vi "Select Comms Method.vi"(8 "Error In":errorcluster) -> (0 "Error Out":errorcluster, 3 "User DOne":bool)   [LabVIEW 2014]
uses:
  Application Support/Stop Button/SubVI/Get Stop Button Status.vi
  Application Support/Front Panel/Window In Front/Bring Caller to Front.vi
  Settings File/SubVI/Load Connection Type.vi
  Settings File/SubVI/Load Serial Baud Rate.vi
  Settings File/SubVI/Save Connection Type.vi
  Settings File/SubVI/Save Baud Rate.vi
  Controls/Telemetry Connection Type.ctl
  Aircraft Information/Sub VI/Set Aircraft Information.vi
  Aircraft Information/Controls/Aircraft Mode.ctl
  Aircraft Information/Controls/Base Mode.ctl
  Aircraft Information/Controls/Drone Information.ctl
  Controls/Telemetry Serial Baud Rate.ctl
  GUI Design/Buttons/Standard button.ctl
panel:
  in  "VISA resource name":refnum<visa-resource-name>
  in  "Baud Rate":T1=enum."115200"
  in  "Connection Type":T2
  out "String":string="COMMUNICATION METHOD"
  in  "Done":T3
  in  "Join Mission":bool
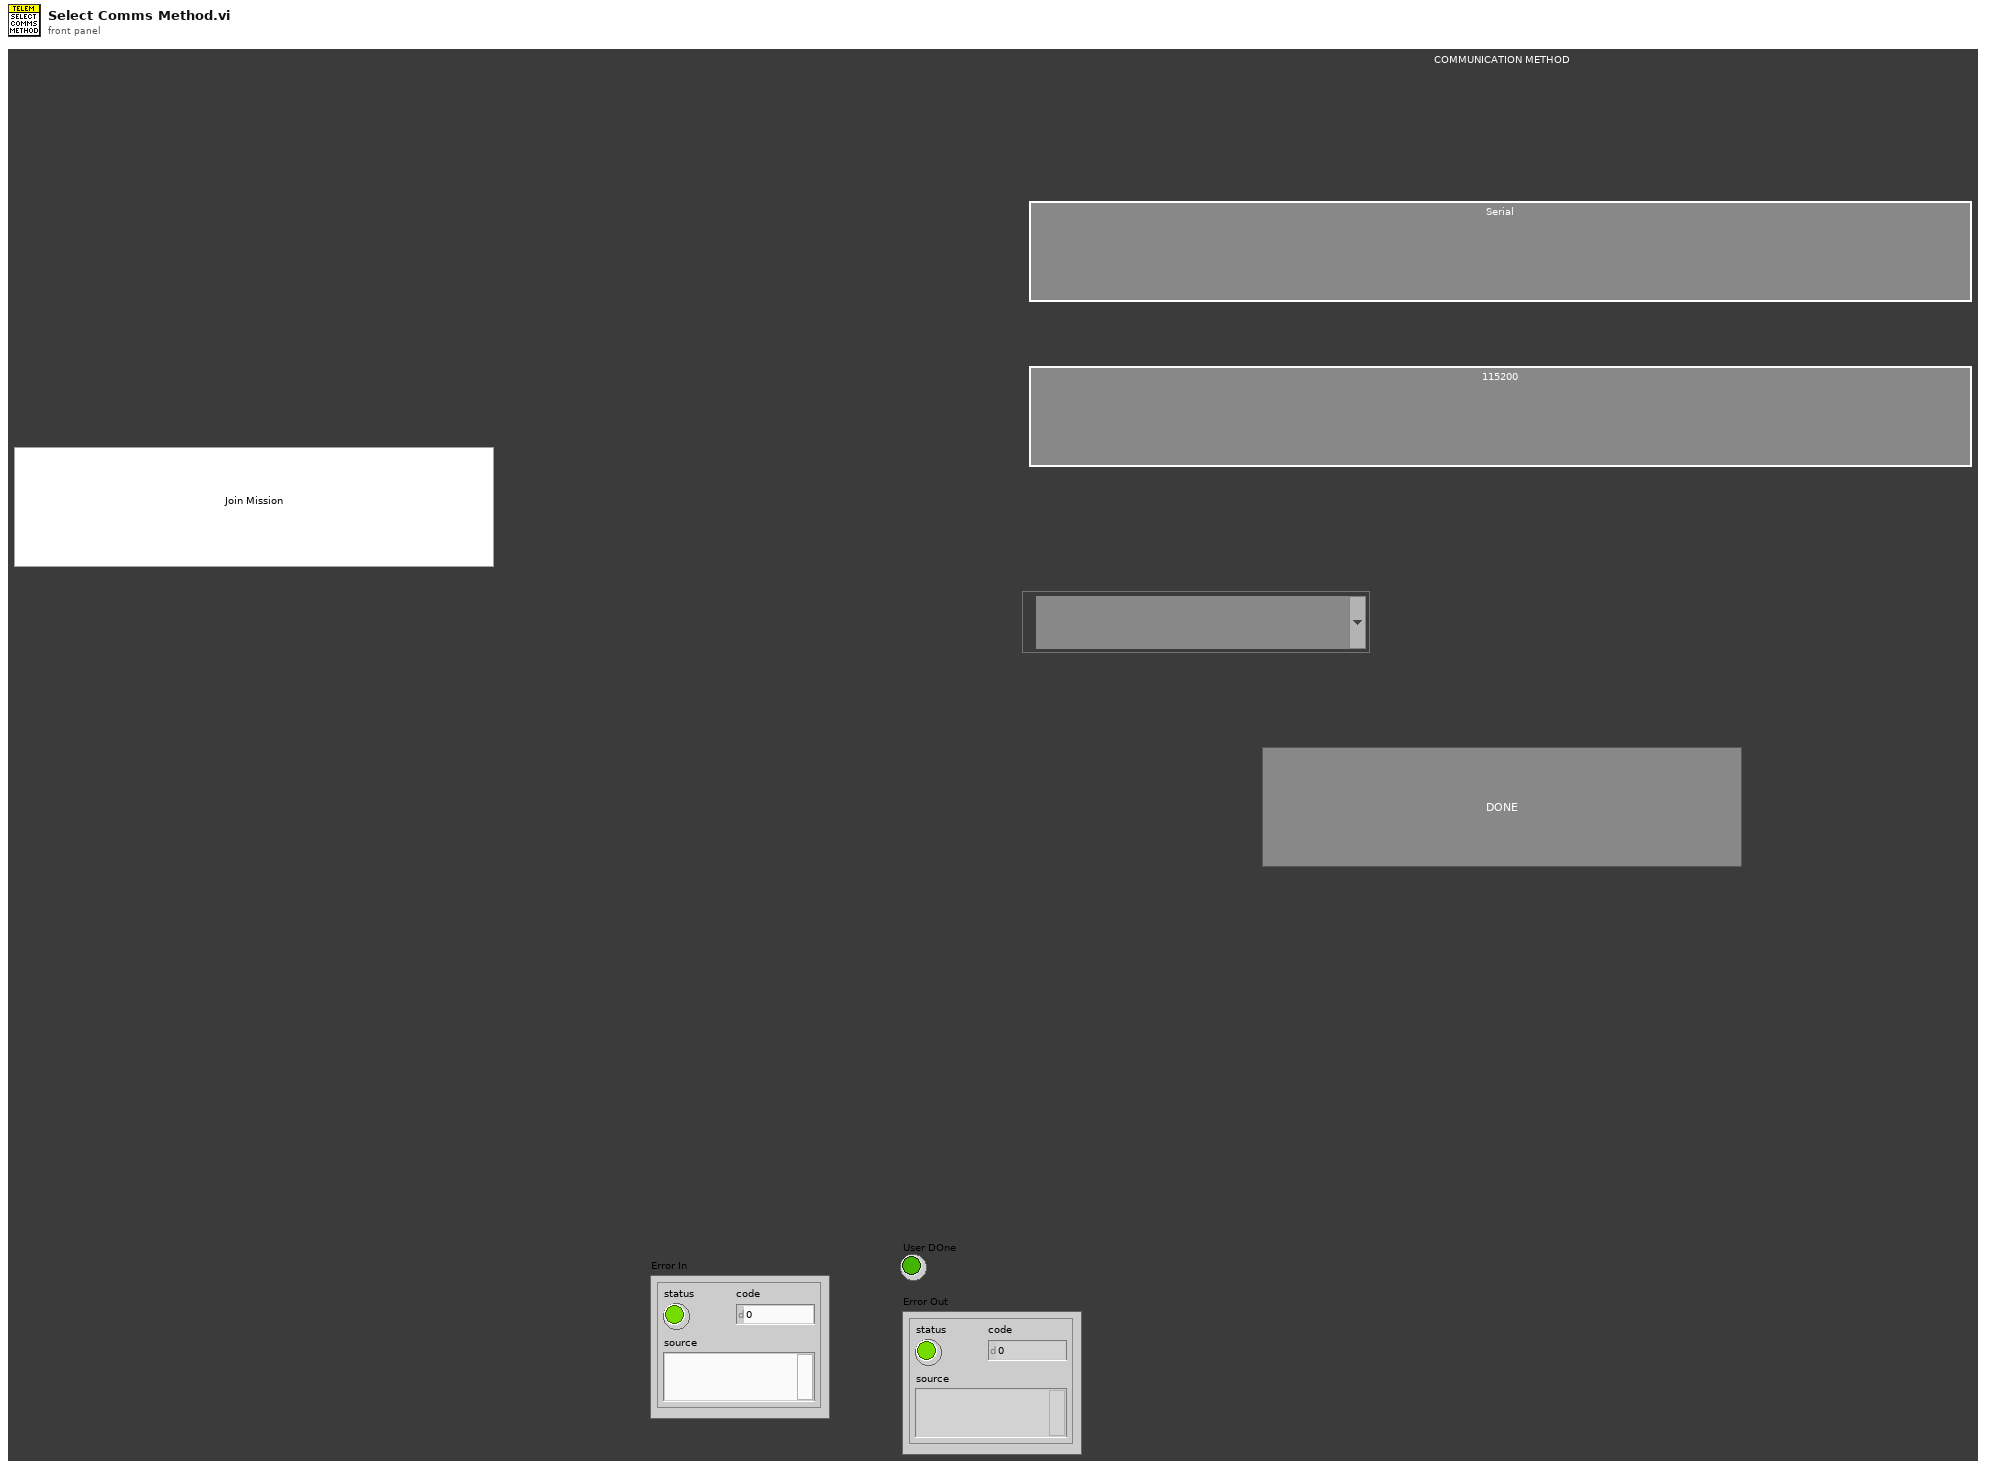
[diagram p1: front panel]
types:
  T1 = typedef "Telemetry Serial Baud Rate.ctl" = enum16{"9600", "38400", "57600", "115200"}
  T2 = typedef "Telemetry Connection Type.ctl" = enum16{"Serial", "UDP", "TCP"}
  T3 = typedef "Standard button.ctl" = bool
  T4 = typedef "Drone Information.ctl" = cluster{"Heart Beat":bool, "Aircraft ID":u8, "Tag ID":string, "System Status":string, "Base Mode":T5, "Armed/Disarmed":bool, "Battery Voltage":dbl, "Control Mode":T6, "Initialisation":u8, "Heart Beat Status":bool, "Mode":string, "Mission Uploaded":bool}
  T5 = typedef "Base Mode.ctl" = cluster{"Custom Mode":bool, "Test Enabled":bool, "Autonomous Mode":bool, "Guided Mode":bool, "Stabilization Enabled":bool, "HIL Enabled":bool, "Manual Mode":bool, "Arm":bool}
  T6 = typedef "Aircraft Mode.ctl" = enum16{"Loiter", "Stabalise", "Failsafe", "Emergency Stop"}
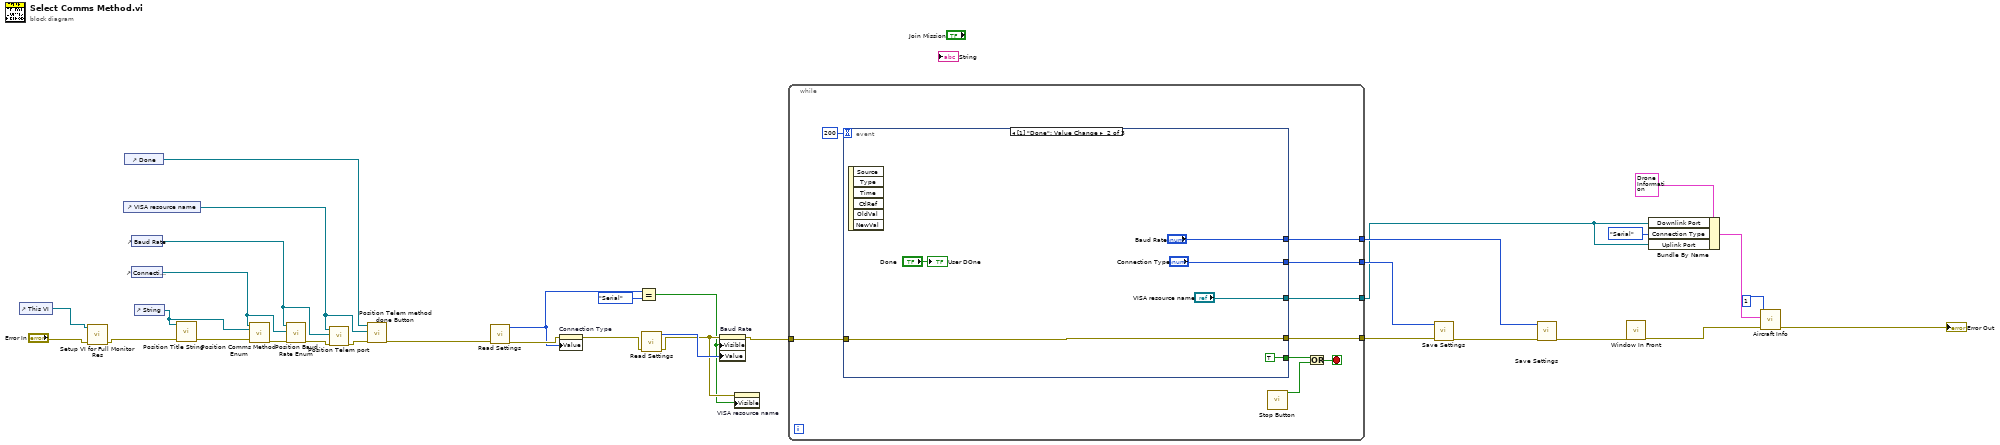
[diagram p0: block diagram]
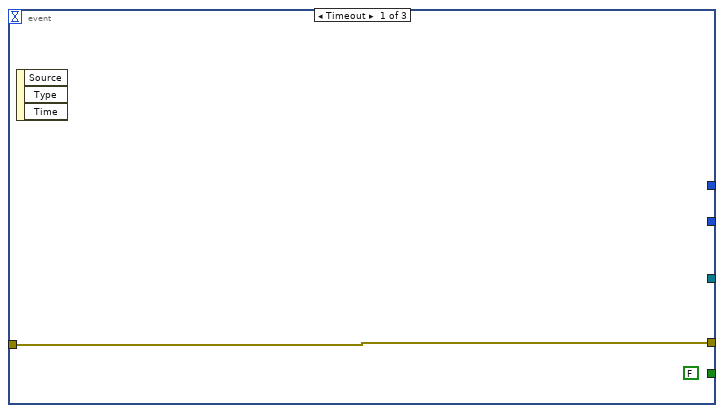
[diagram p2: hidden frame]
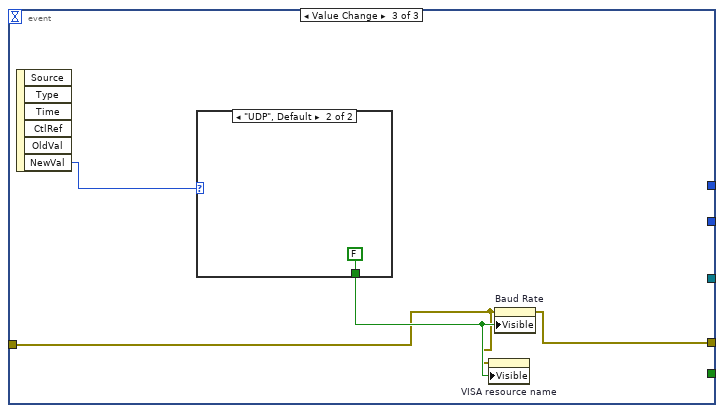
[diagram p3: hidden frame]
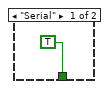
[diagram p4: hidden frame]
diagram:
  n1 = control-ref of="This VI"() -> (w31:refnum<vi>)
  n2 = call "Setup VI for Full Monitor Res.vi"("Error In"="Error In", "This VI"=w31) -> ("Error Out"=w33:errorcluster)  [unwired: 8 in, 1 out]
  n3 = control-ref of="VISA resource name"() -> (w1:refnum<vi>)
  n4 = control-ref of="Done"() -> (w28:refnum<vi>)
  n5 = control-ref of="Baud Rate"() -> (w2:refnum<vi>)
  n6 = control-ref of="Connection Type"() -> (w26:refnum<vi>)
  n7 = control-ref of="String"() -> (w29:refnum<vi>)
  n8 = call "Position Title String.vi"("error in (no error)"=w33, "String Ref"=w29) -> ("error out"=w30:errorcluster)  [unwired: 9 in]
  n9 = call "Position Comms Method Enum.vi"("error in (no error)"=w30, "Previous String"=w29, "Country Enum"=w26) -> ("error out"=w27:errorcluster)  [unwired: 8 in]
  n10 = call "Position Baud Rate Enum.vi"("error in (no error)"=w27, "Previous enum"=w26, "Baud rate enum"=w2) -> ("error out"=w4:errorcluster)  [unwired: 8 in]
  n11 = call "Position Telem port.vi"("error in (no error)"=w4, "comms enum"=w2, "Visa Ref"=w1) -> ("error out"=w3:errorcluster)  [unwired: 8 in]
  n12 = call "Position Telem method done Button.vi"("error in (no error)"=w3, "port enum"=w1, "Button Ref"=w28) -> ("error out"=w24:errorcluster)  [unwired: 8 in]
  n13 = call-poly "Read Settings.vi"("Error In"=w24) -> ("error out"=w23:errorcluster, "Connection Type"=w15:T2)  [unwired: 9 in]
  n14 = property on="Connection Type" class="Enum (strict)"(error in=w23, "Value"=w15) -> (error out=w22:errorcluster)  [unwired: 1 in, 1 out]
  n15 = Equal?(x=w15, y=Telemetry_Connection_Type."Serial") -> (x = y?=w5:bool)
  n16 = call-poly "Read Settings.vi"("Error In"=w22) -> ("error out"=w13:errorcluster, "Baud Rate"=w21:T1)  [unwired: 9 in]
  n17 = property on="Baud Rate" class="Enum (strict)"(error in=w13, "Visible"=w5, "Value"=w21) -> (error out=w25:errorcluster)  [unwired: 1 in, 1 out]
  n18 = property on="VISA resource name" class="VISAName"(error in=w13, "Visible"=w5) -> ()  [unwired: 1 in, 2 out]
  n19 = while {
    tunnel: w25 -> [w39]
    tunnel: [w38] -> w20
    tunnel: [w36] -> w16
    tunnel: [w35] -> w17
    tunnel: [w34] -> w6
    stop <- w41 stop-if-true
    n20 = event shown="[1] \"Done\": Value Change" {
      selector: _ -> [_ _ _]
      dyn-events: _ -> [_ _ _]
      timeout: 200 -> [_ _ _]
      tunnel: [_ TRUE ("x") _] -> w40
      tunnel: w39 -> [w43 w49 w50]
      tunnel: [w43 w49 w52] -> w38
      tunnel: [_ "Connection Type" _] -> w36
      tunnel: [_ "Baud Rate" _] -> w35
      tunnel: [_ "VISA resource name" _] -> w34
      event Timeout {
        (unwired) FALSE ("x")
        n21 = event-data() -> ()  [unwired: 1 in, 3 out]
      }
      event Value Change {
        n22 = event-data() -> ()  [unwired: 1 in, 6 out]
        "User DOne" <- "Done"
      }
      event Value Change {
        n23 = event-data() -> ("NewVal"=w53:T2)  [unwired: 1 in, 5 out]
        n24 = case shown="\"UDP\", Default" w53 {
          tunnel: [TRUE ("Visible") FALSE ("Visible")] -> w51
          frame "Serial" {
          }
          frame "UDP", Default {
          }
        }
        n25 = property on="VISA resource name" class="VISAName"(error in=w50, "Visible"=w51) -> ()  [unwired: 1 in, 2 out]
        n26 = property on="Baud Rate" class="Enum (strict)"(error in=w50, "Visible"=w51) -> (error out=w52:errorcluster)  [unwired: 1 in, 1 out]
      }
    }
    n27 = call-poly "Stop Button.vi"() -> ("Stop ButtonOut"=w42:bool)  [unwired: 10 in, 1 out]
    n28 = Or(x=w40, y=w42) -> (x .or. y?=w41:bool)
  }
  n29 = call-poly "Save Settings.vi"("Error In"=w20, "Connection Type"=w16) -> ("error out"=w19:errorcluster)  [unwired: 9 in]
  n30 = call-poly "Save Settings.vi"("Error In"=w19, "Baud Rate"=w17) -> ("error out"=w18:errorcluster)  [unwired: 9 in]
  n31 = call-poly "Window In Front.vi"("Error In"=w18) -> ("Error Out"=w9:errorcluster)  [unwired: 10 in]
  n32 = Bundle By Name(cluster=T4 {"Heart Beat"=FALSE, "Aircraft ID"=0, "Tag ID"="", "System Status"="", "Base Mode"={"Custom Mode"=FALSE, "Test Enabled"=FALSE, "Autonomous Mode"=FALSE, "Guided Mode"=FALSE, "Stabilization Enabled"=FALSE, "HIL Enabled"=FALSE, "Manual Mode"=FALSE, "Arm"=FALSE}, "Armed/Disarmed"=FALSE, "Battery Voltage"=0.0, "Control Mode"=enum."Stabalise", "Initialisation"=0, "Heart Beat Status"=FALSE, "Mode"="", "Mission Uploaded"=FALSE} ("Aircraft Information In"), "Downlink Port"=w6, "Connection Type"=Telemetry_Connection_Type."Serial", "Uplink Port"=w6) -> (w11:T4)
  n33 = call-poly "Aircraft Info.vi"("Error In"=w9, 10:w11, "Aircraft Information In"=u8 1 ("Aircraft ID")) -> ("Error Out"=→"Error Out":errorcluster)  [unwired: 7 in, 1 out]
